vi "Exemple - AsyncSum.vi"() -> ()   [LabVIEW 2016]
uses:
  Library/DemoSkeleton/DemoSkeleton.lvlib
panel:
  in  "B":i32=2
  in  "A":i32=1
  out "Sum":i64
  # "+"
  # "="
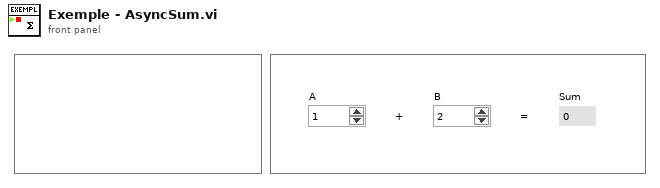
[diagram p1: front panel]
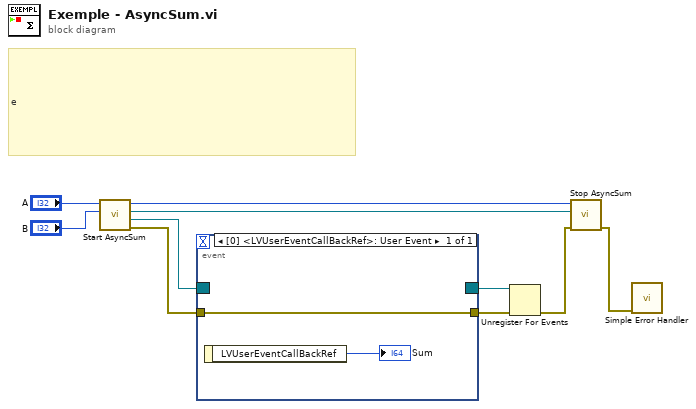
[diagram p0: block diagram]
diagram:
  # "e"
  n1 = call "Start AsyncSum.vi"("B"="B", "A"="A") -> ("error out"=w6:errorcluster, "AsyncSum Event Register"=w5:refnum<event-registration>, "LVUserEvent CallBack Reference"=w3:refnum<user-event>, "Handle"=w4:u64)  [unwired: 6 in]
  n2 = event shown="[0] <LVUserEventCallBackRef>: User Event" {
    selector: w5 -> [_]
    dyn-events: [_] -> w10
    timeout: _ -> [_]
    tunnel: w6 -> [w12]
    tunnel: [w12] -> w9
    event User Event {
      n3 = event-data() -> ("LVUserEventCallBackRef"=→"Sum":i64)  [unwired: 1 in]
    }
  }
  n4 = Unregister For Events(event registration refnum=w10, error in=w9) -> (error out=w2:errorcluster)
  n5 = call "Stop AsyncSum.vi"("error in (no error)"=w2, "LVUserEventCallBackRef"=w3, "Handle"=w4) -> ("error out"=w1:errorcluster)  [unwired: 8 in]
  n6 = call <vilib>:"Simple Error Handler.vi"("error in (no error)"=w1) -> ()  [unwired: 4 in, 5 out]
